vi "Configure Frequency Cable.vi"(0 "VISA resource name":refnum<visa-resource-name>, 5 "frequency (100 Hz)":u16(ring) items=["100 Hz", "120 Hz", "1 kHz", "10 kHz", "20 kHz (option 002 ONLY)", "100 kHz"], 7 "line frequency (60 Hz)":u16(ring)=60 items=["50 Hz", "60 Hz"], 9 "cable length (0 m)":u16(ring) items=["0 m", "1 m", "2 m", "4 m"], 11 "error in (no error)":errorcluster) -> (4 "VISA resource name out":refnum<visa-resource-name>, 15 "error out":errorcluster)   [LabVIEW 2016, in "Agilent 4263X.lvlib"]
doc: "This VI configures the test frequency, the power line frequency and the cable length."
uses:
  <instrlib>/Agilent 4263X/Agilent 4263X.lvlib
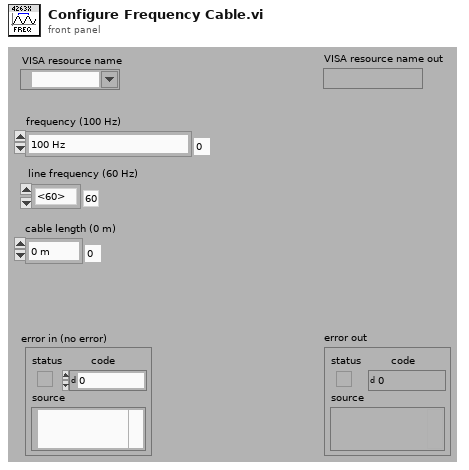
[diagram p1: front panel]
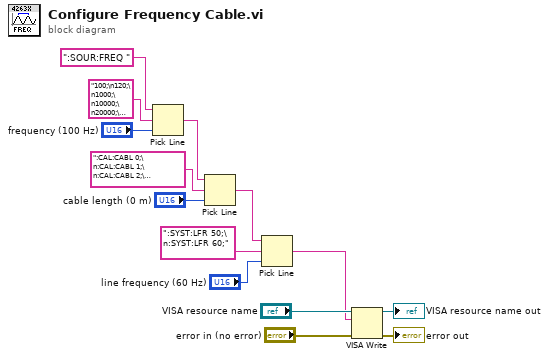
[diagram p0: block diagram]
diagram:
  n1 = Pick Line(string ("")=":SOUR:FREQ ", multi-line string="100;\n120;\n1000;\n10000;\n20000;\n100000;", line index="frequency (100 Hz)") -> (output string=w7:string)
  n2 = Pick Line(string ("")=w7, multi-line string=":CAL:CABL 0;\n:CAL:CABL 1;\n:CAL:CABL 2;\n:CAL:CABL 4;", line index="cable length (0 m)") -> (output string=w4:string)
  n3 = Pick Line(string ("")=w4, multi-line string=":SYST:LFR 50;\n:SYST:LFR 60;", line index="line frequency (60 Hz)") -> (output string=w1:string)
  n4 = VISA Write(VISA resource name="VISA resource name", write buffer=w1, error in (no error)="error in (no error)") -> (VISA resource name out=→"VISA resource name out":refnum<visa-resource-name>, error out=→"error out":errorcluster)  [unwired: 1 out]
